vi "TDT-Set Sys Mode.vi"(0 "Data":T2={"TTankX"=refnum, "TDevAccX"=refnum, "LastTime"=0.0, "error"={"status"=FALSE, "code"=0, "source"=""}, "Block Name"="", "Circuit Tag"="", "Tank Name"="", "NumTicks"=0, "LastTick"=0.0, "Idle?"=FALSE, "Wait (ms)"=1000, "LastArtf"=0.0, "LastTosc"=0.0}, 7 "NewMode":T1, 11 "error in (no error)":errorcluster) -> (15 "error out":errorcluster)   [LabVIEW 2015]
uses:
  TDT Interface Data.ctl
  TDT-Sys Mode Enum.ctl
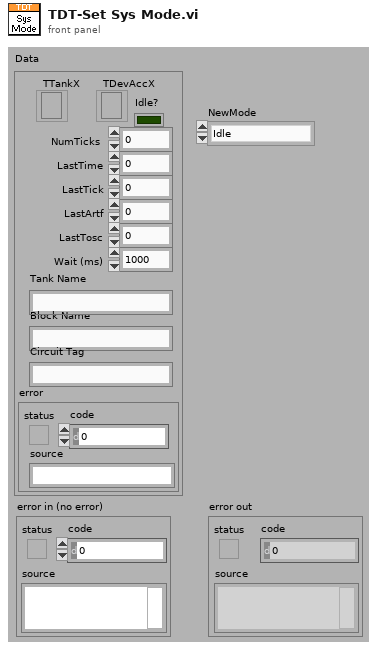
[diagram p1: front panel]
types:
  T1 = typedef "TDT-Sys Mode Enum.ctl" = enum16{"Idle", "Standby", "Preview", "Record"}
  T2 = typedef "TDT Interface Data.ctl" = cluster{"TTankX":refnum<k7>, "TDevAccX":refnum<k7>, "LastTime":dbl, "error":errorcluster, "Block Name":string, "Circuit Tag":string, "Tank Name":string, "NumTicks":i32, "LastTick":dbl, "Idle?":bool, "Wait (ms)":u32, "LastArtf":dbl, "LastTosc":dbl}
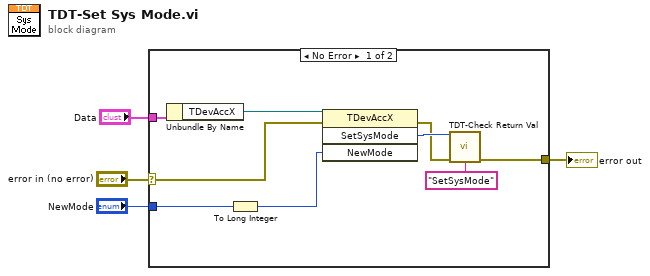
[diagram p0: block diagram]
diagram:
  n1 = case shown="No Error" "error in (no error)" {
    selector: "error in (no error)" -> [w9 w14]
    tunnel: [w8 w14] -> w3
    tunnel: "Data" -> [w7 _]
    tunnel: "NewMode" -> [w6 _]
    frame No Error {
      n2 = Unbundle By Name(w7) -> ("TDevAccX"=w13:refnum<k7>)
      n3 = To Long Integer(number=w6) -> (32bit integer=w5:i32)
      n4 = invoke class="TDevAccX" method="SetSysMode"(reference=w13, error in=w9, "NewMode"=w5) -> (error out=w11:errorcluster, "SetSysMode"=w12:i32)  [unwired: 1 in, 2 out]
      n5 = call "TDT-Check Return Val.vi"("Return Val"=w12, "error in (no error)"=w11, "source"="SetSysMode" ("Message")) -> ("error out"=w8:errorcluster)  [unwired: 12 in]
    }
    frame Error {
    }
  }
  "error out" <- w3
